vi "showCursorLabel.vi"(6 "Cursor Properties":T1={"Horizontal Line?"=TRUE, "Vertical Line?"=TRUE, "Timestamp"=enum."at BOTTOM", "time format (%H:%M:%S)"="%H:%M:%S", "size"=2, "font"={"Font Name"="Arial", "Size"=16, "Strikeout?"=FALSE, "Italic?"=FALSE, "Underline?"=FALSE, "Outline?"=FALSE, "Shadow"=FALSE, "Bold?"=FALSE}, "alignment(left, top)"={"Horizontal"=enum."center", "Vertical"=enum."center"}, "TextFormat"="%3$s\\n%2$.2f"} {"size" min=1 max=50}, 7 "Picture in":picture, 8 "error in (no error)":errorcluster, 9 "XY Values":cluster{"X":dbl, "X":dbl}, 10 "origin":cluster{"x":i16, "y":i16}, 11 "QControl_Graph in":refnum<class "QControl_Graph.lvclass">) -> (0 "error out":errorcluster, 3 "QControl_Graph out":refnum<class "QControl_Graph.lvclass">, 5 "Picture out":picture)   [LabVIEW 2017, in "QControl_Graph.lvclass"]
uses:
  QControl_Graph.lvclass
  C:/Program Files (x86)/National Instruments/LabVIEW 2017/vi.lib/QSI/QControls/QControl Classes/WaveformGraph/WaveformGraph.lvclass
  Cursor Properties.ctl
  Font.ctl
  Alignment.ctl
  Alignment.Horizontal.ctl
  Alignment.Vertical.ctl
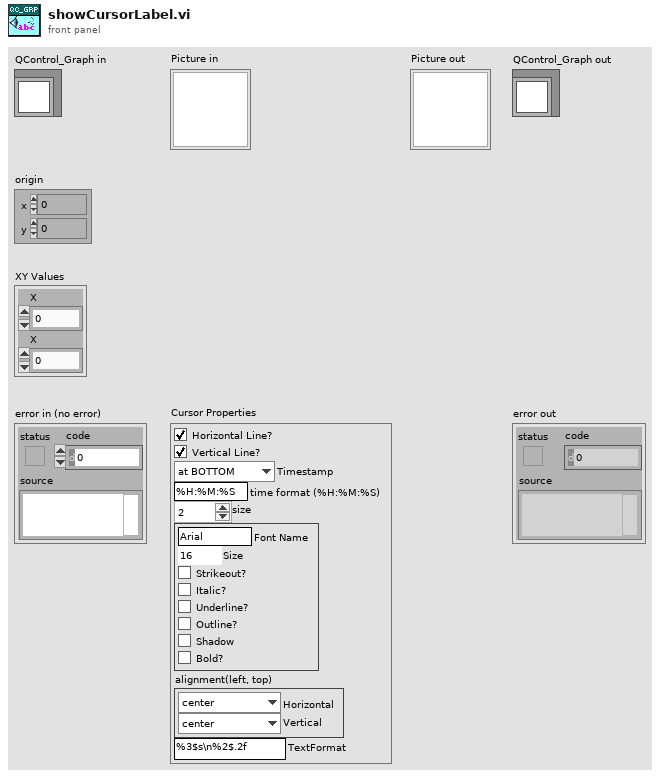
[diagram p1: front panel]
types:
  T1 = typedef "QControl_Graph.lvclass/Cursor Properties.ctl" = cluster{"Horizontal Line?":bool, "Vertical Line?":bool, "Timestamp":enum16{"at TOP", "at BOTTOM", "none"}, "time format (%H:%M:%S)":string, "size":i16, "font":T2, "alignment(left, top)":T3, "TextFormat":string}
  T2 = typedef "QControl_Graph.lvclass/Font.ctl" = cluster{"Font Name":string, "Size":i16, "Strikeout?":bool, "Italic?":bool, "Underline?":bool, "Outline?":bool, "Shadow":bool, "Bold?":bool}
  T3 = typedef "QControl_Graph.lvclass/Alignment.ctl" = cluster{"Horizontal":T4, "Vertical":T5}
  T4 = typedef "QControl_Graph.lvclass/Alignment.Horizontal.ctl" = enum16{"left", "center", "right"}
  T5 = typedef "QControl_Graph.lvclass/Alignment.Vertical.ctl" = enum16{"top", "center", "bottom"}
  T6 = enum16{"User-specified Font", "Application Font", "System Font", "Dialog Font"}
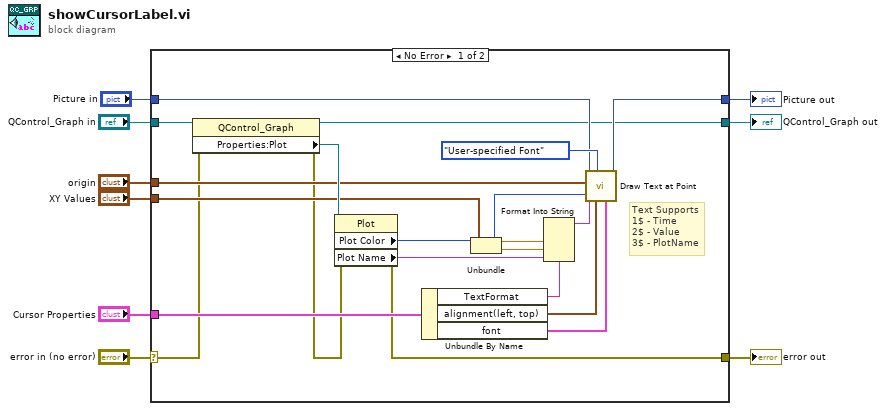
[diagram p0: block diagram]
diagram:
  n1 = case shown="No Error" "error in (no error)" {
    selector: "error in (no error)" -> [w19 w32]
    tunnel: [w10 w32] -> w8
    tunnel: [w11 w31] -> w6
    tunnel: "QControl_Graph in" -> [w29 w31]
    tunnel: "Cursor Properties" -> [w28 _]
    tunnel: "origin" -> [w24 _]
    tunnel: "XY Values" -> [w21 _]
    tunnel: "Picture in" -> [w13 w30]
    tunnel: [w12 w30] -> w1
    frame No Error {
      # "Text Supports\n1$ - Time\n2$ - Value\n3$ - PlotName"
      n2 = property class="QControl_Graph"(reference=w29, error in=w19) -> (reference out=w11:refnum<class "QControl_Graph.lvclass">, error out=w18:errorcluster, "Properties:Plot"=w26:refnum<vi>)
      n3 = property class="Plot"(reference=w26, error in=w18) -> (error out=w10:errorcluster, "Plot Color"=w25:u32, "Plot Name"=w17:string)  [unwired: 1 out]
      n4 = Unbundle By Name(w28) -> ("TextFormat"=w16:string, "alignment(left, top)"=w15:T3, "font"=w27:T2)
      n5 = Unbundle(w21) -> ("X"=w23:dbl, "X"=w22:dbl)
      n6 = Format Into String(format string=w16, w23, w22, w17) -> (resulting string=w20:string)  [unwired: 2 in, 1 out]
      n7 = call <vilib>:"Draw Text at Point.vi"("[user-specified font]"=w27, "text color(black)"=w25, "desired font(Application)"=T6."User-specified Font", "text"=w20, "alignment(left, top)"=w15, "origin"=w24, "picture"=w13) -> ("new picture"=w12:picture)  [unwired: 3 in, 1 out]
    }
    frame Error {
    }
  }
  "error out" <- w8
  "QControl_Graph out" <- w6
  "Picture out" <- w1
